vi "Compare Direction.vi"(10 "Current Angle":dbl, 11 "Destination Angle":dbl) -> (2 "CW(-1)/CCW(1)":dbl, 3 "Angle to Next Destination":dbl)   [LabVIEW 2011]
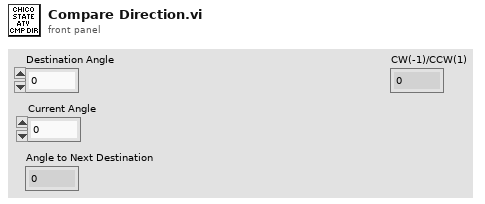
[diagram p1: front panel]
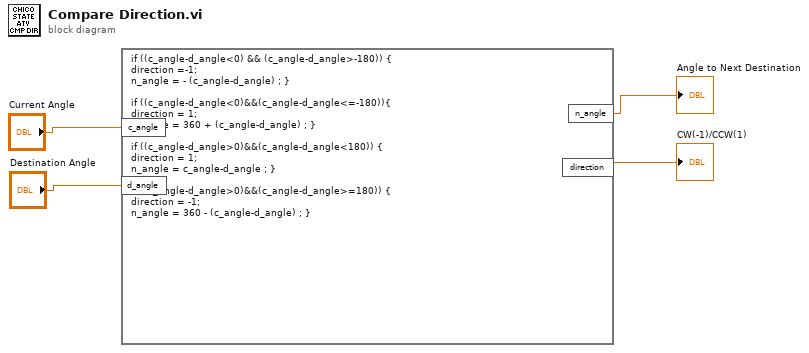
[diagram p0: block diagram]
diagram:
  n1 = formula code="if ((c_angle-d_angle<0) && (c_angle-d_angle>-180)) {\ndirection =-1;\nn_angle = - (c_angle-d_angle) ; }\n\nif ((c_angle-d_angle<0)&&(c_angle-d_angle<=-180)){\ndirection = 1;\nn_angle = 360 + (c_angle-d_angle) ; }\n\nif ((c_angle-d_angle>0)&&(c_angle-d_angle<180)) {\ndirection = 1;\nn_angle = c_angle-d_angle ; }\n\nif ((c_angle-d_angle>0)&&(c_angle-d_angle>=180)) {\ndirection = -1;\nn_angle = 360 - (c_angle-d_angle) ; }"("c_angle"="Current Angle", "d_angle"="Destination Angle") -> ("n_angle"=→"Angle to Next Destination":dbl, "direction"=→"CW(-1)/CCW(1)":dbl)
